vi "Kepco cfg enable output.vi"(8 "error in (no error)":errorcluster {"code" format="%.0x"}, 9 "Simulation":T1, 10 "Channel parsed command info":T2, 11 "input cluster":refnum<class "KepcoBOP.lvclass">) -> (0 "error out":errorcluster, 2 "new commands":string, 3 "output cluster":refnum<class "KepcoBOP.lvclass">)   [LabVIEW 2013, in "KepcoBOP.lvclass"]
uses:
  KepcoBOP.lvclass
  Shared/Device Driver/channel parsed cmd cluster.ctl
  shared/OnOffTypeDef.ctl
  KepcoBOP.lvclass/KepcoBOP.ctl
  shared/CompressAndUpdate(Poly)/CompressAndUpdate(Enum).vi
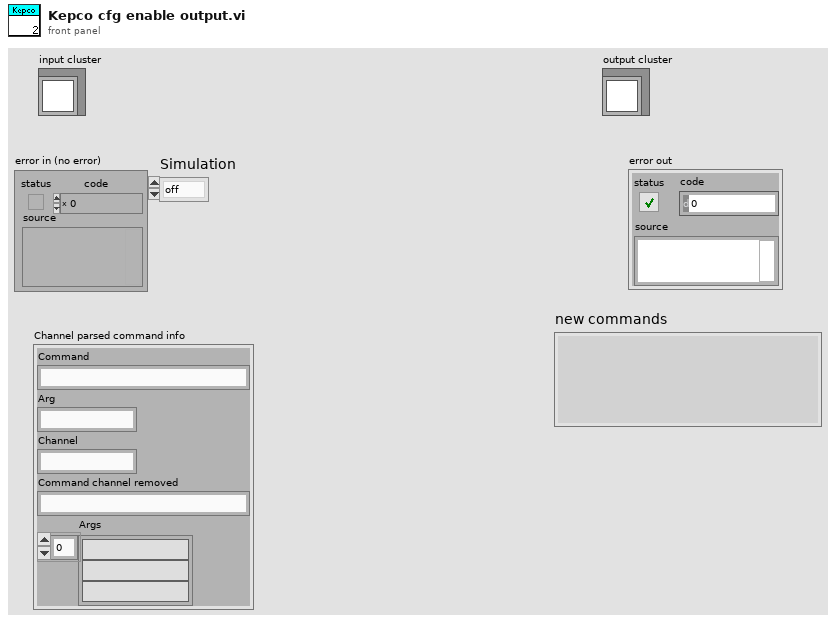
[diagram p1: front panel]
types:
  T1 = typedef "OnOffTypeDef.ctl" = enum16{"off", "on"}
  T2 = typedef "channel parsed cmd cluster.ctl" = cluster{"Command":string, "Arg":string, "Channel":string, "Command channel removed":string, "Args":string[]}
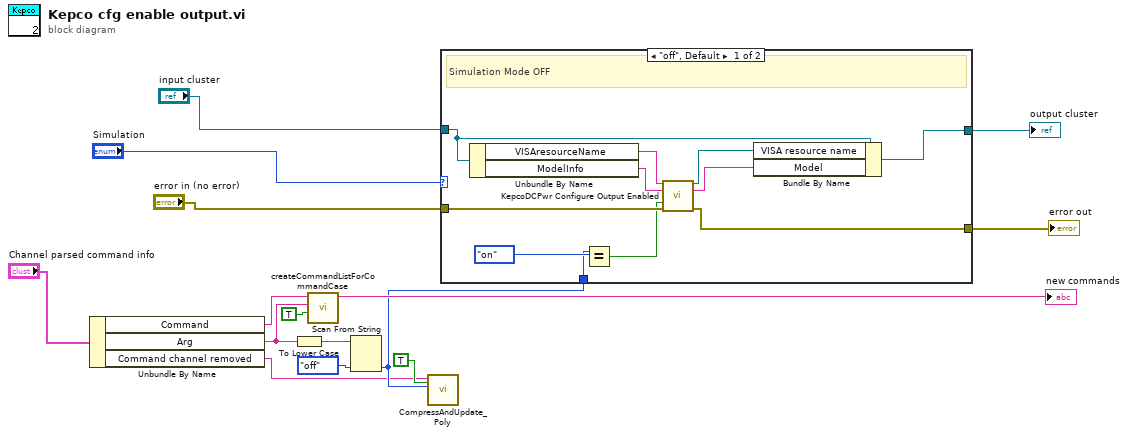
[diagram p0: block diagram]
diagram:
  n1 = Unbundle By Name("Channel parsed command info") -> ("Command"=w14:string, "Arg"=w3:string, "Command channel removed"=w1:string)
  n2 = To Lower Case(string=w3) -> (all lower case string=w5:string)
  n3 = call "createCommandListForCommandCase.vi"("immediate Check (only once)"=TRUE, "setvalue"=w3, "command"=w14) -> ("new commands"=→"new commands":string)  [unwired: 8 in]
  n4 = Scan From String(input string=w5, default 1=enum16{"off", "on"}."off") -> (output 1=w2:enum16{"off", "on"})  [unwired: 3 in, 3 out]
  n5 = call-poly "CompressAndUpdate_Poly.vi"("force CVT update (false)"=TRUE ("force CVT update"), "enum variant"=w2, "command or variable name"=w1) -> ()  [unwired: 8 in, 1 out]
  n6 = case shown="\"off\", Default" "Simulation" {
    tunnel: [w18 w27] -> w9
    tunnel: "input cluster" -> [w26 w28]
    tunnel: "error in (no error)" -> [w20 w27]
    tunnel: [w25 w28] -> w10
    tunnel: w2 -> [w23 _]
    frame "off", Default {
      # "Simulation Mode OFF"
      n7 = Unbundle By Name(w26) -> ("VISAresourceName"=w22:string, "ModelInfo"=w21:string)
      n8 = Equal?(x=w23, y=enum16{"off", "on"}."on") -> (x = y?=w19:bool)
      n9 = call "KepcoDCPwr Configure Output Enabled.vi"("VISA Session"=w22, "Model In"=w21, "Input enabled (True)"=w19, "error in (no error)"=w20) -> ("VISA Session Out"=w16:refnum<visa-resource-name>, "Model Out"=w17:string, "error out"=w18:errorcluster)  [unwired: 9 in]
      n10 = Bundle By Name(cluster=w26, "VISA resource name"=w16, "Model"=w17) -> (w25:refnum<class "KepcoBOP.lvclass">)
    }
    frame "on" {
      # "Simulation Mode ON"
    }
  }
  "output cluster" <- w10
  "error out" <- w9
